vi "Controller_Main.vi"(8 "error in (no error)":errorcluster) -> (0 "error out":errorcluster)   [LabVIEW 2020]
uses:
  #typedef_ControllerQueue_States.ctl
  User Interface/#typedef_UserInterface_Data.ctl
  User Interface/Cmd_enum.ctl
  User Interface/#typedef_Parameters_cluster.ctl
  User Interface/BaudRate_enum.ctl
  Data Base/#typedef_DataBase.ctl
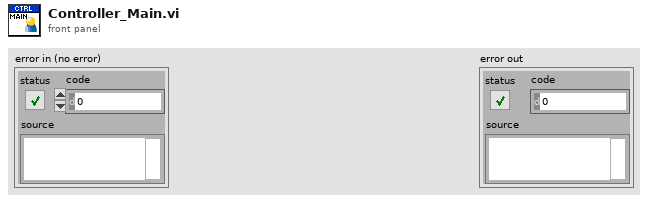
[diagram p1: front panel]
types:
  T1 = typedef "#typedef_ControllerQueue_States.ctl" = enum16{"Obtain", "GetRef", "Enqueue", "EnqueueAtOpp", "GetStatus", "Flush", "Release"}
  T2 = typedef "Cmd_enum.ctl" = enum16{"Init", "PrintChart", "Connect", "Disconnect", "ReadData", "Exit"}
  T3 = typedef "#typedef_UserInterface_Data.ctl" = cluster{"Cmd":T2, "Param":T4, "Temperature":dbl, "Logs":string}
  T4 = typedef "#typedef_Parameters_cluster.ctl" = cluster{"Stop":bool, "Connect":bool, "Disconnect":bool, "Port COM":refnum<visa-resource-name>, "Baud rate":T5}
  T5 = typedef "BaudRate_enum.ctl" = enum16{"115200", "9600"}
  T6 = typedef "#typedef_DataBase.ctl" = cluster{"Cmd":enum16{"Idle", "WriteLog", "Exit"}, "Temperature":dbl, "Logs":string}
  T7 = typedef "#typedef_Controller_Data.ctl" = cluster{"Cmd":enum16{"Idle", "PrintChart", "SendToDB", "Exit"}, "Temperature":dbl, "Logs":string}
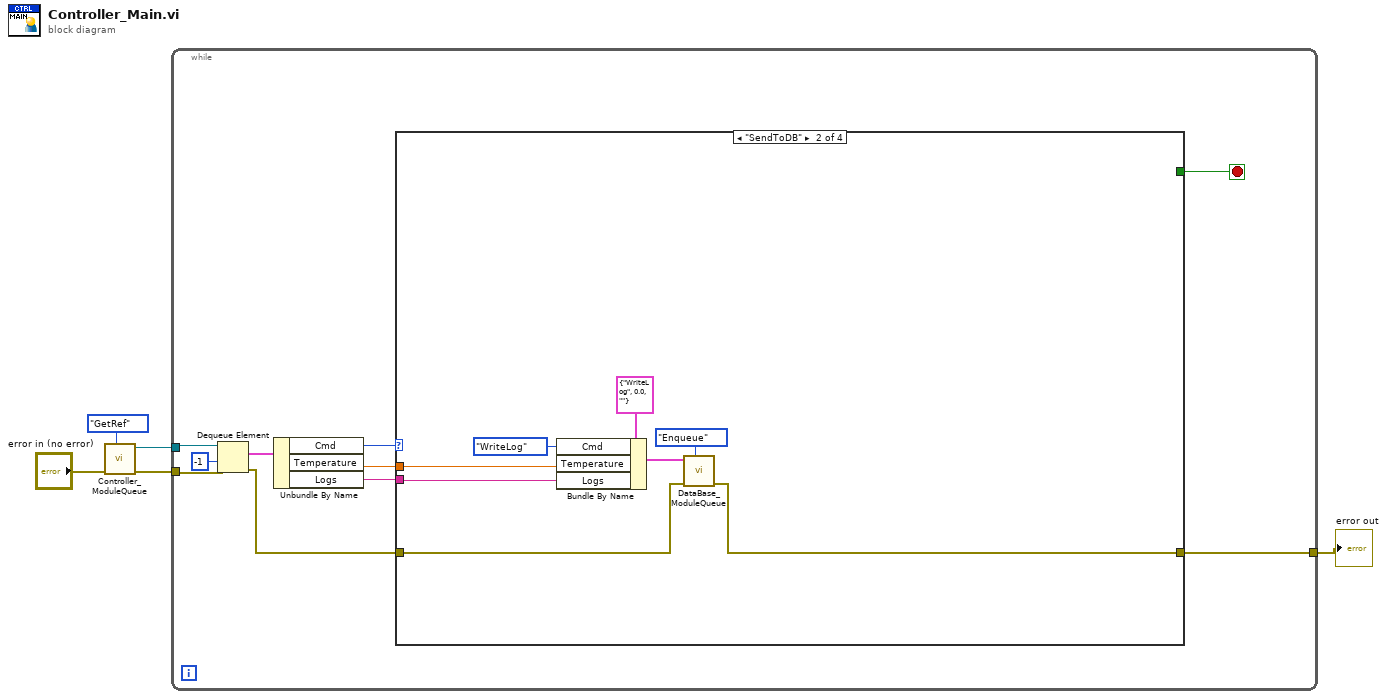
[diagram p0: block diagram]
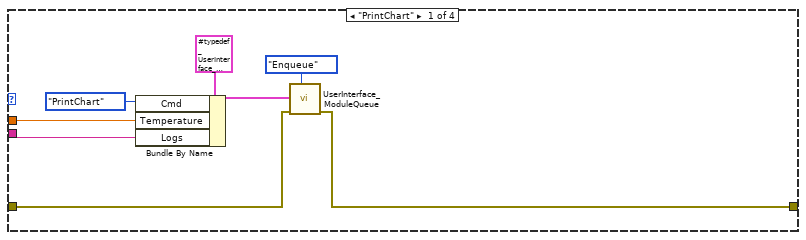
[diagram p2: hidden frame]
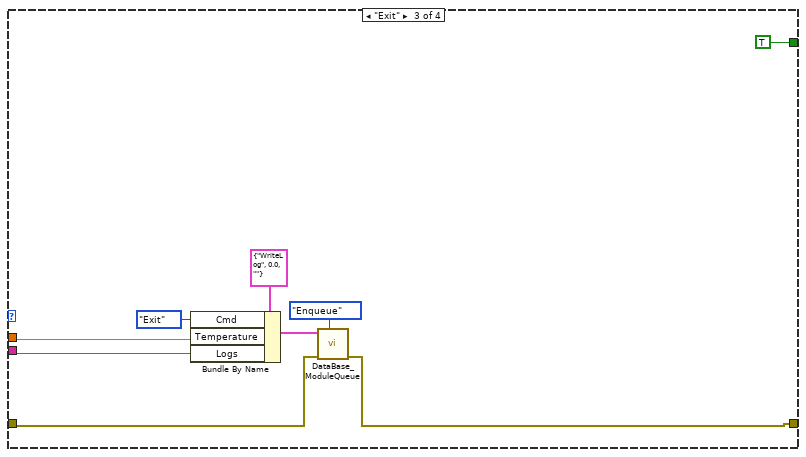
[diagram p3: hidden frame]
diagram:
  n1 = call "Controller_ModuleQueue.vi"(7:#typedef_ControllerQueue_States."GetRef", "error in (no error)"="error in (no error)") -> ("error out"=w5:errorcluster, "queue out"=w2:refnum<queue>)  [unwired: 7 in, 1 out]
  n2 = while {
    tunnel: w5 -> [w13]
    tunnel: w2 -> [w12]
    tunnel: [w7] -> w1
    stop <- w9 stop-if-true
    n3 = Dequeue Element(queue=w12, timeout in ms (-1)=-1, error in (no error)=w13) -> (element=w15:T7, error out=w8:errorcluster)  [unwired: 2 out]
    n4 = Unbundle By Name(w15) -> ("Cmd"=w11:enum16{"Idle", "PrintChart", "SendToDB", "Exit"}, "Temperature"=w10:dbl, "Logs"=w6:string)
    n5 = case shown="\"SendToDB\"" w11 {
      tunnel: w10 -> [w17 w25 w33 _]
      tunnel: [_ _ TRUE _] -> w9
      tunnel: w8 -> [w22 w28 w35 w41]
      tunnel: [w21 w27 w36 w41] -> w7
      tunnel: w6 -> [w16 w26 w34 _]
      frame "PrintChart" {
        n6 = Bundle By Name(cluster=T3 {"Cmd"=enum."Init", "Param"={"Stop"=FALSE, "Connect"=FALSE, "Disconnect"=FALSE, "Port COM"="", "Baud rate"=enum."115200"}, "Temperature"=0.0, "Logs"=""} ("DataIn"), "Cmd"=Cmd_enum."PrintChart", "Temperature"=w17, "Logs"=w16) -> (w20:T3)
        n7 = call "UserInterface_ModuleQueue.vi"(7:#typedef_ControllerQueue_States."Enqueue", "error in (no error)"=w22, "DataIn"=w20) -> ("error out"=w21:errorcluster)  [unwired: 6 in, 2 out]
      }
      frame "SendToDB" {
        n8 = Bundle By Name(cluster=T6 {"Cmd"=enum."WriteLog", "Temperature"=0.0, "Logs"=""} ("DB Data"), "Cmd"=enum16{"Idle", "WriteLog", "Exit"}."WriteLog", "Temperature"=w25, "Logs"=w26) -> (w29:T6)
        n9 = call "DataBase_ModuleQueue.vi"(7:#typedef_ControllerQueue_States."Enqueue", "error in (no error)"=w28, "DB Data"=w29) -> ("error out"=w27:errorcluster)  [unwired: 6 in, 2 out]
      }
      frame "Exit" {
        n10 = Bundle By Name(cluster=T6 {"Cmd"=enum."WriteLog", "Temperature"=0.0, "Logs"=""} ("DB Data"), "Cmd"=enum16{"Idle", "WriteLog", "Exit"}."Exit", "Temperature"=w33, "Logs"=w34) -> (w37:T6)
        n11 = call "DataBase_ModuleQueue.vi"(7:#typedef_ControllerQueue_States."Enqueue", "error in (no error)"=w35, "DB Data"=w37) -> ("error out"=w36:errorcluster)  [unwired: 6 in, 2 out]
      }
      frame "Idle" {
      }
    }
  }
  "error out" <- w1
